vi "CalculateStartupMetrics.vi"(10 "Channel":T5, 11 "DataSets":T1[](array[typedef])) -> (2 "Startup features":T4, 3 "Features":T6[](array[typedef]))   [LabVIEW 2017, in "McsaStartupAnalysis.lvlib"]
uses:
  <vilib>/addons/InsightCM/Devices/Shared/Mcsa/McsaStartupAnalysis/McsaStartupAnalysis.lvlib
  <vilib>/addons/InsightCM/Devices/Shared/Mcsa/McsaStartupAnalysis/controls/StartupFeature.ctl
  <vilib>/addons/InsightCM/Devices/Shared/Mcsa/McsaStartupAnalysis/controls/ChannelForStartup.ctl
  <vilib>/addons/InsightCM/Devices/Shared/Mcsa/McsaStartupAnalysis/controls/MotorInfo.ctl
  <vilib>/addons/InsightCM/Devices/Shared/Common/DataEvent/controls/DataSet.ctl
  <vilib>/addons/InsightCM/MessageBus/Base/controls/DataSetMetadata.ctl
  <vilib>/addons/InsightCM/MessageBus/Base/controls/KeyValuePair.ctl
  <vilib>/addons/InsightCM/Utilities/Analysis/MCSA/McsaAnalysisFunctions.lvlib
  <vilib>/addons/InsightCM/Devices/Shared/Common/DataEvent/DataEvent.lvlib
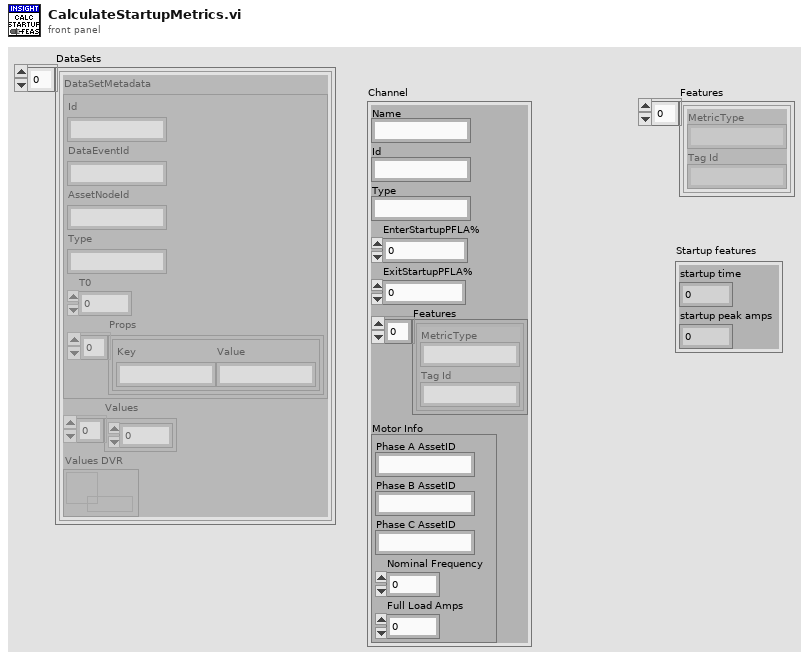
[diagram p1: front panel]
types:
  T1 = typedef "DataEvent.lvlib/DataSet.ctl" = cluster{"DataSetMetadata":T2, "Values":sgl[], "Values DVR":refnum<data-value>}
  T2 = typedef "DataSetMetadata.ctl" = cluster{"Id":string, "DataEventId":string, "AssetNodeId":string, "Type":string, "T0":i64, "Props":T3[]}
  T3 = typedef "KeyValuePair.ctl" = cluster{"Key":string, "Value":string}
  T4 = cluster{"startup time":dbl, "startup peak amps":dbl}
  T5 = typedef "McsaStartupAnalysis.lvlib/ChannelForStartup.ctl" = cluster{"Name":string, "Id":string, "Type":string, "EnterStartupPFLA%":dbl, "ExitStartupPFLA%":dbl, "Features":T6[], "Motor Info":T7}
  T6 = typedef "McsaStartupAnalysis.lvlib/StartupFeature.ctl" = cluster{"MetricType":string, "Tag Id":string}
  T7 = typedef "McsaStartupAnalysis.lvlib/MotorInfo.ctl" = cluster{"Phase A AssetID":string, "Phase B AssetID":string, "Phase C AssetID":string, "Nominal Frequency":dbl, "Full Load Amps":dbl}
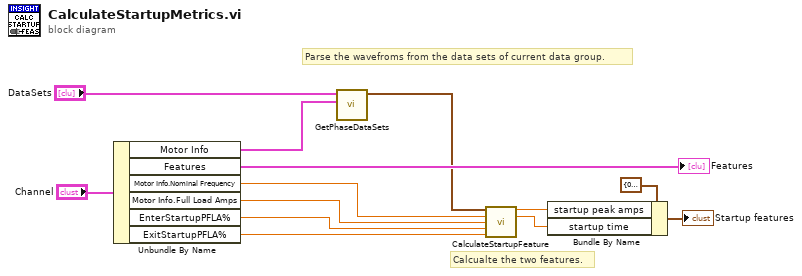
[diagram p0: block diagram]
diagram:
  # "Calcualte the two features."
  # "Parse the wavefroms from the data sets of current data group."
  n1 = Unbundle By Name("Channel") -> ("Motor Info"=w4:T7, "Features"=→"Features":T6[], "Motor Info.Nominal Frequency"=w2:dbl, "Motor Info.Full Load Amps"=w1:dbl, "EnterStartupPFLA%"=w3:dbl, "ExitStartupPFLA%"=w11:dbl)
  n2 = call <vilib>:"GetPhaseDataSets.vi"("Motor Info"=w4, "DataSets"="DataSets") -> ("ValidPhaseDataSets"=w5:waveform(sgl)[])  [unwired: 9 in]
  n3 = call <vilib>:"CalculateStartupFeature.vi"("current waveforms"=w5, "nameplate frequency"=w2, "Full Load Amps"=w1, "start trigger level [%]"=w3, "stop trigger level [%]"=w11) -> ("startup peak amps"=w9:dbl, "startup time"=w8:dbl)  [unwired: 8 in, 1 out]
  n4 = Bundle By Name(cluster=T4 {"startup time"=0.0, "startup peak amps"=0.0} ("Startup features"), "startup peak amps"=w9, "startup time"=w8) -> (→"Startup features":T4)
